vi "FindBestPath.vi"(8 "error in (no error)":errorcluster, 11 "OccupancyMap in":refnum<class "OccupancyMap.lvclass">) -> (0 "error out":errorcluster, 1 "found":bool, 2 "path":cluster{"X":dbl, "Y":dbl}[](array[cluster]), 3 "OccupancyMap out":refnum<class "OccupancyMap.lvclass">)   [LabVIEW 2014, in "OccupancyMap.lvclass"]
uses:
  <userlib>/AdvancedDataStructures/ClassBased/Applications/Occupancy/OccupancyMap/OccupancyMap.lvclass
  <userlib>/AdvancedDataStructures/ClassBased/Graph/SearchMethod.ctl
  <userlib>/AdvancedDataStructures/ClassBased/Applications/Occupancy/Cell/Cell.lvclass
  <userlib>/AdvancedDataStructures/ClassBased/Applications/Occupancy/OccupancyMap/OccupancyMap.lvclass/OccupancyMap.ctl
  <userlib>/AdvancedDataStructures/ClassBased/Graph/Graph.lvclass
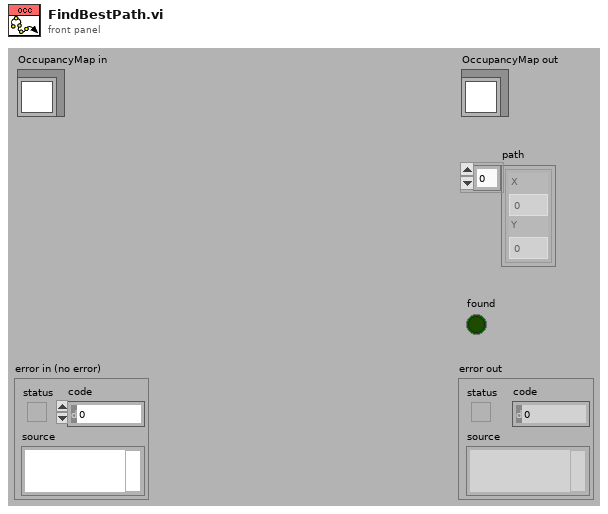
[diagram p1: front panel]
types:
  T1 = typedef "Graph.lvlib/Graph.lvclass/SearchMethod.ctl" = enum16{"Breadth (First)", "Depth (First)", "Best First", "Breadth (Best)", "Depth (Best)"}
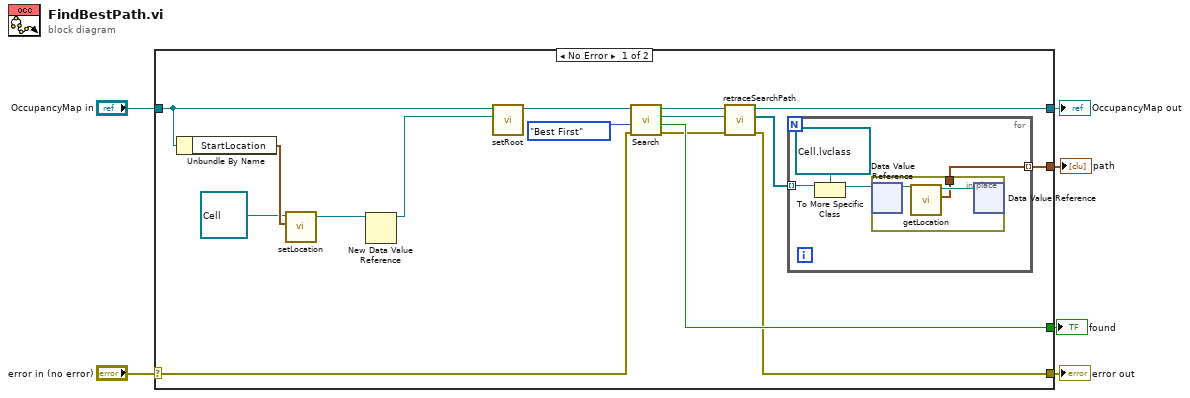
[diagram p0: block diagram]
diagram:
  n1 = case shown="No Error" "error in (no error)" {
    selector: "error in (no error)" -> [w22 w31]
    tunnel: [w10 w31] -> w5
    tunnel: [w13 w30] -> w3
    tunnel: "OccupancyMap in" -> [w17 w30]
    tunnel: [w21 _] -> w2
    tunnel: [w9 _] -> w1
    frame No Error {
      n2 = Unbundle By Name(w17) -> ("StartLocation"=w19:cluster{"X":dbl, "Y":dbl})
      n3 = call <userlib>:"setLocation.vi"("Location"=w19, "Cell in"=refnum<class "Cell.lvclass"> refnum ("Cell.lvclass")) -> ("Cell out"=w8:refnum<class "Cell.lvclass">)  [unwired: 8 in, 1 out]
      n4 = New Data Value Reference(data value=w8) -> (data value reference=w7:refnum<data-value>)  [unwired: 1 in, 1 out]
      n5 = call <userlib>:"setRoot.vi"("Root"=w7, "Graph in"=w17) -> ("Graph out"=w16:refnum<class "OccupancyMap.lvclass">)  [unwired: 8 in, 1 out]
      n6 = call <userlib>:"Search.vi"("error in (no error)"=w22, "SearchMethod"=SearchMethod."Best First", "Graph in"=w16) -> ("error out"=w11:errorcluster, "found"=w21:bool, "Node"=w15:refnum<data-value>, "Graph out"=w14:refnum<class "OccupancyMap.lvclass">)  [unwired: 5 in]
      n7 = call <userlib>:"retraceSearchPath.vi"("error in (no error)"=w11, "GoalNode"=w15, "Graph in"=w14) -> ("error out"=w10:errorcluster, "SearchPath"=w12:refnum<data-value>[], "Graph out"=w13:refnum<class "OccupancyMap.lvclass">)  [unwired: 6 in]
      n8 = for {
        tunnel: w12 -> [w26] mode=indexing
        tunnel: [w23] -> w9 mode=indexing
        n9 = To More Specific Class(target class=refnum<data-value> refnum ("data value reference"), reference=w26) -> (specific class reference=w24:refnum<data-value>)  [unwired: 1 in, 1 out]
        n10 = in-place {
          in-place-border: [w27] -> w23
          n11 = in-place-dvr #1(w24) -> (w29:refnum<class "Cell.lvclass">)  [unwired: 1 out]
          n12 = call <userlib>:"getLocation.vi"("Cell in"=w29) -> ("Location"=w27:cluster{"X":dbl, "Y":dbl}, "Cell out"=w28:refnum<class "Cell.lvclass">)  [unwired: 8 in, 1 out]
          n13 = in-place-dvr #1(w28) -> ()  [unwired: 2 out]
        }
      }
    }
    frame Error {
    }
  }
  "error out" <- w5
  "OccupancyMap out" <- w3
  "path" <- w1
  "found" <- w2
